vi "MDF4 Write Data to Stream (Double).vi"(7 "path in":path, 8 "Error In":errorcluster, 9 "data":dbl[](array[numeric]), 10 "chan_count":u64, 11 "Stream Reference in":i64) -> (0 "Error Out":errorcluster, 3 "Stream Reference out":i64)   [LabVIEW 2019, in "MD4Logger Engine.lvlib"]
uses:
  MD4Logger Engine.lvlib
  <vilib>/Utility/error.llb/Error Cluster From Error Code.vi
  <vilib>/ErrorRing/Error Ring.xnode
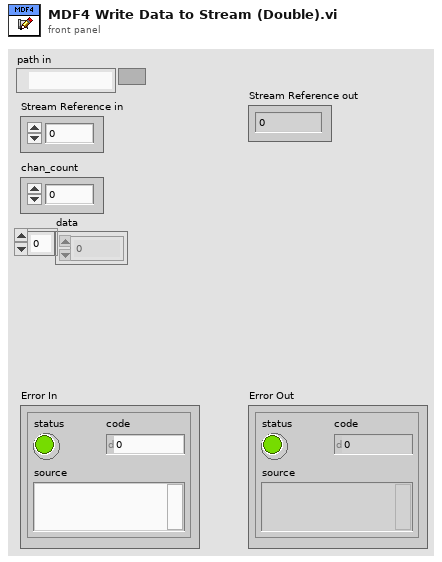
[diagram p1: front panel]
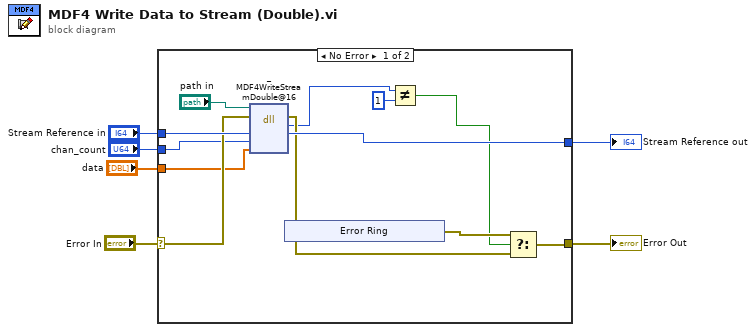
[diagram p0: block diagram]
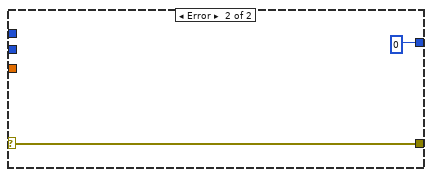
[diagram p2: hidden frame]
diagram:
  n1 = case shown="No Error" "Error In" {
    selector: "Error In" -> [w17 w25]
    tunnel: "Stream Reference in" -> [w18 _]
    tunnel: [w13 w25] -> w4
    tunnel: [w16 i64 0 ("m4")] -> w3
    tunnel: "chan_count" -> [w15 _]
    tunnel: "data" -> [w7 _]
    frame No Error {
      n2 = dll-call lib="C:/Users/Hovhannes/Desktop/MD4Logger/Source/Engine/DLL/WriterExample.dll" fn="_MDF4WriteStreamDouble@16"(path in="path in", error in=w17, "DStream"=w18, "chan_count"=w15, "data"=w7) -> (error out=w12:errorcluster, "return type"=w10:i32, "DStream"=w16:i64)  [unwired: 3 in, 1 out]
      n3 = xnode "Error Ring"() -> ("error out"=w14:errorcluster)
      n4 = Not Equal?(x=w10, y=1) -> (x != y?=w9:bool)
      n5 = Select(t=w14, s=w9, f=w12) -> (s? t:f=w13:errorcluster)
    }
    frame Error {
    }
  }
  "Error Out" <- w4
  "Stream Reference out" <- w3
